vi "macro_LinearSystemLoop_FlyWheel_Execute.vi"() -> ()   [LabVIEW 2019, in "Trajectory_Library.lvlib"]
uses:
  Trajectory_Library.lvlib
  Enum/DCMOTOR_TYPES_ENUM.ctl
panel:
  in  "Velocity (Rad/Sec)\n(PV)":dbl
  in  "Velocity (Rad/Sec)\nSetpoint (SP)":dbl
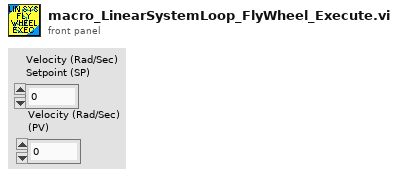
[diagram p1: front panel]
types:
  T1 = typedef "Trajectory_Library.lvlib/DCMOTOR_TYPES_ENUM.ctl" = enum16{"CIM", "AndyMark 9015", "Andy Mark RS 775 125", "Bag", "BaneBots RS 550", "BaneBots RS 775", "Falcon 500", "Mini CIM", "NEO", "NEO 550", "Romi BuiltIn", "Vex 775 Pro", "Snow Blower AM 2235A", "Bosch Seat AM 3493"}
  T2 = typedef "Trajectory_Library.lvlib/LINEAR_SYSTEM_ID_FLYWHEEL_MODEL.ctl" = cluster{"DCMOTOR_TYPES":T1, "Num Motors":i32, "Gearing":dbl, "MOI kgm2":dbl}
  T3 = typedef "Trajectory_Library.lvlib/LINEAR_SYSTEM_LOOP_FLYWHEEL_CTRL_PARAMS.CTL" = cluster{"Vel Model Std Dev Rad/Sec":dbl, "Vel Meas Std Dev Rad/Sec":dbl, "Vel Ctrl Tol Rad/Sec":dbl, "Max Ctrl Out V":dbl}
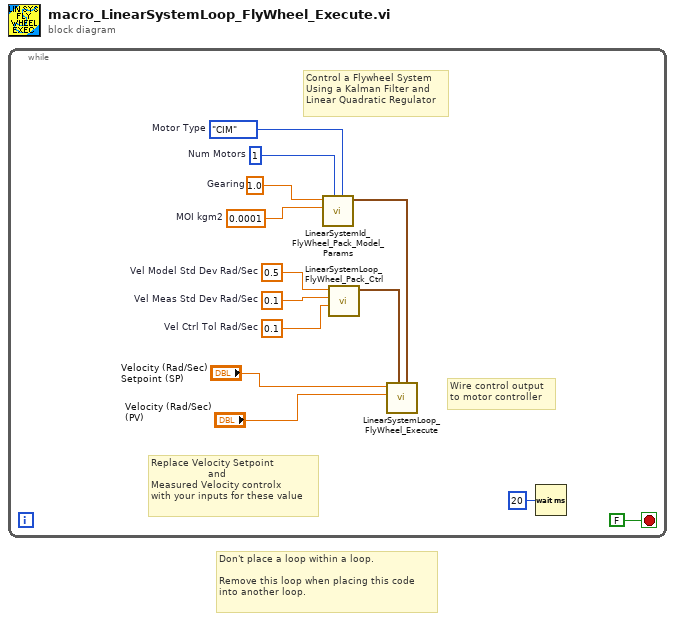
[diagram p0: block diagram]
diagram:
  # "Don't place a loop within a loop.\n \nRemove this loop when placing this code\ninto another loop."
  n1 = while {
    stop <- FALSE stop-if-true
    w3 = 0.5  # Vel Model Std Dev Rad/Sec
    w4 = 0.1  # Vel Meas Std Dev Rad/Sec
    w5 = 0.1  # Vel Ctrl Tol Rad/Sec
    w10 = 1.0  # Gearing
    w11 = 0.0001  # MOI kgm2
    w12 = 1  # Num Motors
    w13 = DCMOTOR_TYPES_ENUM."CIM"  # Motor Type
    # "Wire control output\nto motor controller"
    # "Replace Velocity Setpoint \n                   and \nMeasured Velocity controlx\nwith your inputs for these value"
    # "Control a Flywheel System\nUsing a Kalman Filter and \nLinear Quadratic Regulator"
    n2 = call "LinearSystemId_FlyWheel_Pack_Model_Params.vi"("DCMOTOR_TYPES"=w13, "Num Motors"=w12, "MOI kgm2"=w11, "Gearing"=w10) -> ("FlyWheelSim_Model _Params"=w7:T2)  [unwired: 7 in]
    n3 = call "LinearSystemLoop_FlyWheel_Pack_Ctrl.vi"("Vel Ctrl Tol Rad/Sec"=w5, "Vel Meas Std Dev Rad/Sec"=w4, "Vel Model Std Dev Rad/Sec"=w3) -> ("LinearSystemLoop_FlyWheel_Ctrl_Params"=w6:T3)  [unwired: 8 in]
    n4 = call "LinearSystemLoop_FlyWheel_Execute.vi"("FlyWheelSim_Model _Params"=w7, "LinearSystem_FlyWheel_Ctrl_Params"=w6, "Velocity (Rad/Sec)\n(PV)"="Velocity (Rad/Sec)\n(PV)", "Velocity (Rad/Sec)\nSetpoint (SP)"="Velocity (Rad/Sec)\nSetpoint (SP)") -> ()  [unwired: 5 in, 3 out]
    n5 = Wait (ms)(milliseconds to wait=u32 20) -> ()  [unwired: 1 out]
  }
